vi "Asana_Get.vi"() -> ()   [LabVIEW 2016]
uses:
  <vilib>/httpClient/LabVIEWHTTPClient.lvlib
panel:
  out "Status":string="Idle"
  out "Posting":bool
  out "Body":string="{\"data\":[{\"id\":485255656454849,\"name\":\"Figure out useful API\"},{\"id\":485254540535137,\"name\":\"Figure out useful API\"},{\"id\":483708705076284,\"name\":\"Panther Express Order: CDWG-UPS Battery and Surge protect\"},{\"id\":483695768647078,\"name\":\"Panther Express Order: Grainger - Lascar PS and Scissors\"},{\"id\":483186151754105,\"name\":\"Create a VI that will write a file from a publisher account\"},{\"id\":483194240106048,\"name\":\"Updated CV\"},{\"id\":482695055398718,\"name\":\"Panther Express Order: McMaster - screws, scissors, kapton\"},{\"id\":482610217212443,\"name\":\"Panther Express Order: CDWG-UPS\"},{\"id\":407585611130158,\"name\":\"Damaged items reported in spreadsheet\"},{\"id\":480655848280849,\"name\":\"Panther Express Order: McMaster, Stool for PPMS-DR\"},{\"id\":477959774752493,\"name\":\"Panther Express Order: Grainger stool, etc \"},{\"id\":469638907892082,\"name\":\"QiLi-STO-111-20171024\"},{\"id\":468583209739952,\"name\":\"Panther Express Order: Asylum Research - MFP3D Head Cable\"},{\"id\":466476349857321,\"name\":\"Panther Express Order: Grainger - Roach Kill\"},{\"id\":457225516744036,\"name\":\"Panther Express Order: Grainger - 80/20 Special, Wipers, Tags\"},{\"id\":454524704921360,\"name\":\"Make sure CrystalDiskInfo is running on all of your computers\"},{\"id\":452970255761186,\"name\":\"Panther Express Order: Supra-box, pad, pen, etc\"},{\"id\":450812542170439,\"name\":\"Panther Express Order: B&H, Eneloop 24 batteries \"},{\"id\":446045519104814,\"name\":\"Consider updating your project progress\"},{\"id\":444259581739545,\"name\":\"Panther Express Order: B and H\"},{\"id\":444239318532799,\"name\":\"AsanaBot\"},{\"id\":444214864144911,\"name\":\"Panther Express Order: B and H\"},{\"id\":440454660069823,\"name\":\"Consider updating your project progress\"},{\"id\":439961699416282,\"name\":\"Panther Express Order: Trek Inc \"},{\"id\":439870432141290,\"name\":\"Mapping P/Q as administrator\"},{\"id\":436590367663471,\"name\":\"Read my review of this proposal...\"},{\"id\":437423317842248,\"name\":\"Panther Express Order: CDWG\"},{\"id\":437329183636606,\"name\":\"Panther Express Order: B and H\"},{\"id\":436631000244016,\"name\":\"High-res figures\"},{\"id\":436559576756788,\"name\":\"Review of nature comm paper\"},{\"id\":434949292379141,\"name\":\"Consider updating your project progress\"},{\"id\":431940026570584,\"name\":\"Panther Express Order: Digi-Key\"},{\"id\":431925542819742,\"name\":\"Referee response\"},{\"id\":431034812539576,\"name\":\"Yun-Yi Pai: One-Dimensional Nature of Pairing and Superconductivity at the LaAlO$_3$/SrTiO$_3$ Interface\"},{\"id\":429748551490256,\"name\":\"Panther Express Order: Clark Industry\"},{\"id\":429369274315774,\"name\":\"Consider updating your project progress\"},{\"id\":427825096134432,\"name\":\"Panther Express Order: McMaster\"},{\"id\":427691222436037,\"name\":\"Panther Express Order: Grainger\"},{\"id\":427277290178716,\"name\":\"Panther Express Order: DSS Stockroom\"},{\"id\":426355781160522,\"name\":\"Panther Express Order: McMaster\"},{\"id\":425300320621268,\"name\":\"Panther Express Order: Grainger\"},{\"id\":424594916917454,\"name\":\"Panther Express Order: Grainger\"},{\"id\":423850849835180,\"name\":\"Consider updating your project progress\"},{\"id\":421666010658533,\"name\":\"Panther Express Order: Grainger\"},{\"id\":420450292188130,\"name\":\"Panther Express Order: Count on Tool\"},{\"id\":420274285984926,\"name\":\"Panther Express Order: Supra\"},{\"id\":419973503694738,\"name\":\"A Direct Observation of Room-Temperature Stable Magnetism in LaAlO3/SrTiO3 Heterostructures\"},{\"id\":419007200960117,\"name\":\"Give overview for journal club\"},{\"id\":419211939595159,\"name\":\"Consider updating your project progress\"},{\"id\":418633899494665,\"name\":\"Panther Express Order: Supra\"},{\"id\":418460550035164,\"name\":\"Panther Express Order: Grainger\"},{\"id\":417308065082471,\"name\":\"Pai -- One-Dimensional Nature of Pairing and Superconductivity at the LaAlO$_3$/SrTiO$_3$ Interface\"},{\"id\":417251714966828,\"name\":\"Contact chemarxiv and request removal\"},{\"id\":416724750801660,\"name\":\"Panther Express Order: Digikey\"},{\"id\":416595815316983,\"name\":\"Panther Express Order: CDWG\"},{\"id\":341271010416338,\"name\":\"Leiden CF\"},{\"id\":341271010416342,\"name\":\"PPMS2\"},{\"id\":341271010416340,\"name\":\"MFP3D\"},{\"id\":341701327168967,\"name\":\"Al-SQUID-LAO/STO\"},{\"id\":341701327168968,\"name\":\"1D pairing\"},{\"id\":341271010416334,\"name\":\"Terraces dependence\"},{\"id\":341271010416332,\"name\":\"mK-SPM\"},{\"id\":415394130917359,\"name\":\"Panther Express Order: CDWG\"},{\"id\":415362392608675,\"name\":\"Dying Gallowspole \"},{\"id\":414565496145468,\"name\":\"Panther Express Order: Swagelok\"},{\"id\":414560486678095,\"name\":\"Panther Express Order: PowerTronics\"},{\"id\":414320125293616,\"name\":\"Consider updating your project progress\"},{\"id\":414812763297541,\"name\":\"Backing up Rodia and MFP3D2\"},{\"id\":413707812430964,\"name\":\"Panther Express Order: McMaster\"},{\"id\":412918590813922,\"name\":\"Panther Express Order: Grainger\"},{\"id\":412854250028279,\"name\":\"Panther Express Order: CDWG\"},{\"id\":414812763297546,\"name\":\"Reinstall Rambleon\"},{\"id\":411816952648488,\"name\":\"Panther Express Order: B and H\"},{\"id\":411480040793004,\"name\":\"Panther Express Order: Swagelok\"},{\"id\":411050668817382,\"name\":\"Panther Express Order: Supra\"},{\"id\":410849061822813,\"name\":\"DPC_WATCHDOG_VIOLATION on Windows 10\"},{\"id\":409776701454530,\"name\":\"Panther Express Order: Pfeiffer\"},{\"id\":409725261839576,\"name\":\"Consider updating your project progress\"},{\"id\":408932010835224,\"name\":\"Panther Express Order: Grainger\"},{\"id\":408919683676834,\"name\":\"Panther Express Order: Amazon: Temperhum\"},{\"id\":125608329011186,\"name\":\"order compressed helium\"},{\"id\":407773830393582,\"name\":\"Panther Express Order: LDS Vacuum\"},{\"id\":406802063162283,\"name\":\"UPS Managment and Notification\"},{\"id\":406559591036482,\"name\":\"Panther Express Order: CDWG\"},{\"id\":405460834658478,\"name\":\"Consider updating your project progress\"},{\"id\":404688001223643,\"name\":\"Request for source files: ROPP-100843: \"},{\"id\":403046568483305,\"name\":\"Panther Express Order: B and H\"},{\"id\":240014679645070,\"name\":\"321\"},{\"id\":402248496272499,\"name\":\"From colossal magnetoresistance to solar cells: An overview on 66 years of research into perovskites - Wagner - 2017 - physica status solidi (a) - Wiley Online Library\"},{\"id\":402048376624132,\"name\":\"Panther Express Order: Bluetooth and USB hub\"},{\"id\":402043948639390,\"name\":\"Panther Express Order: Mini-Circuits\"},{\"id\":395892811110536,\"name\":\"Erkut's Visit 2017-08-18\"},{\"id\":400906336596665,\"name\":\"Prospects and Applications Near Ferroelectric Quantum Phase Transitions: A Key Issues Review - IOPscience\"},{\"id\":400863128359472,\"name\":\"Consider updating your project progress\"},{\"id\":400471558989507,\"name\":\"Panther Express Order: Grainger\"},{\"id\":399182657074560,\"name\":\"Post-review modification\"},{\"id\":398583205092188,\"name\":\"Quantized chiral edge conduction on reconfigurable domain walls of a magnetic topological insulator\"},{\"id\":395081310173961,\"name\":\"Panther Express Order: NanoAndMore\"},{\"id\":394425995952756,\"name\":\"Panther Express Order: B and H\"},{\"id\":394147578577517,\"name\":\"Consider updating your project progress\"},{\"id\":393741570332048,\"name\":\"Panther Express Order: Fischer Sci\"},{\"id\":393728961490683,\"name\":\"Panther Express Order: Grainger\"},{\"id\":393425861799391,\"name\":\"Loupe glasses\"},{\"id\":393425861799386,\"name\":\"Humidity Sensor\"},{\"id\":389919070479676,\"name\":\"LED strip\"},{\"id\":392966204577369,\"name\":\"Panther Express Order: Grainger\"},{\"id\":389627825545944,\"name\":\"Consider updating your project progress\"},{\"id\":387484035385757,\"name\":\"Optical routing of TI/STO\"},{\"id\":389052060077622,\"name\":\"[1704.00831] Local optical control of ferromagnetism and chemical potential in a topological insulator\"},{\"id\":387348374446247,\"name\":\"Pai - Present at Group Meeting\"},{\"id\":387264140967807,\"name\":\"Panther Express Order: McMaster\"},{\"id\":385840145696294,\"name\":\"Panther Express Order: McMaster\"},{\"id\":384863397073870,\"name\":\"Consider updating your project progress\"},{\"id\":384334139849136,\"name\":\"Panther Express Order: Hard Drives for Levylab\"},{\"id\":384282457934644,\"name\":\"Panther Express Order: McMaster\"},{\"id\":367057474417733,\"name\":\"New PC (MFP3D)\"},{\"id\":364325321406644,\"name\":\"Document discussing thermal expansion and other issues\"},{\"id\":364325321406641,\"name\":\"Vertical holder for microscope at RT\"},{\"id\":340398386241075,\"name\":\"Isolation Transformer\"},{\"id\":326775992935276,\"name\":\"mK SPM group at ETH\"},{\"id\":321962801394065,\"name\":\"\\\"Matrix box\\\" to filter LEMO signals (black and yellow)\"},{\"id\":378962853779249,\"name\":\"misc\"},{\"id\":344607718799273,\"name\":\"2017-05-17 Skype Meeting\"},{\"id\":248358351003361,\"name\":\"Section 1 - Overview \"},{\"id\":298912981556577,\"name\":\"Nano Letters\"},{\"id\":126345791674174,\"name\":\"Make sure the server is online\"},{\"id\":255953270721811,\"name\":\"Is there a way to configure NaNs get stored as -1?\"},{\"id\":234136524959348,\"name\":\"Gallowspole\"},{\"id\":234136523931720,\"name\":\"PPM2 (Misty)\"},{\"id\":102892368894317,\"name\":\"Coupling to Al SQUIDs (w/ Hatridge)\"},{\"id\":193137962305231,\"name\":\"New PC and PXI\"},{\"id\":174316714177126,\"name\":\"noise in non-contact mode\"},{\"id\":16346183834689,\"name\":\"Videos of how to use MFP3D correctly\"},{\"id\":164934741081297,\"name\":\"Check out and summarize datafinder\"},{\"id\":164713499062215,\"name\":\"Send an Email to Zeldov (this week)\"},{\"id\":5715673502818,\"name\":\"Scanning SET measurements of LAO/STO nanowires w/ Shahal Ilani\"},{\"id\":126345791674164,\"name\":\"Web Services\"},{\"id\":5715673502814,\"name\":\"Nano-SQUID measurements of magnetization and spin currents with Eli Zeldov\"},{\"id\":136636634213865,\"name\":\"Humidity sensing and control outside of the enclosure\"},{\"id\":60311354850707,\"name\":\"SQUID Mask\"},{\"id\":106146774472944,\"name\":\"Writing along and across unit cell steps\"},{\"id\":64122220487809,\"name\":\"Contact Nanomag\"},{\"id\":48971181341219,\"name\":\"Driver for mK AFM\"},{\"id\":15150235906125,\"name\":\"24 to 20 pin adapter\"},{\"id\":49727592364466,\"name\":\"characterize any heating from piezos\"},{\"id\":14977236170882,\"name\":\"Au/LAO/STO Structures\"},{\"id\":383650859418411,\"name\":\"PO:\"},{\"id\":382951012845538,\"name\":\"Panther Express Order: McMaster\"},{\"id\":381019968837796,\"name\":\"Panther Express Order: Digikey\"},{\"id\":379898116941267,\"name\":\"Consider updating your project progress\"},{\"id\":379501609976135,\"name\":\"Panther Express Order: Grainger\"},{\"id\":359337230461679,\"name\":\"Panther Express Order: Grainger Special\"},{\"id\":368042101946896,\"name\":\"Panther Express Order: NanoScience\"},{\"id\":383650859418412,\"name\":\"Review:\"},{\"id\":372506422905539,\"name\":\"PhysRevMaterials.1.011601\"},{\"id\":375791389169587,\"name\":\"Consider updating your project progress\"},{\"id\":373555267523795,\"name\":\"Panther Express Order: Quantum Design\"},{\"id\":372521984820550,\"name\":\"Panther Express Order: Mouser\"},{\"id\":372518137565892,\"name\":\"Panther Express Order: CDWG\"},{\"id\":372517342438507,\"name\":\"Panther Express Order: Grainger\"},{\"id\":372516415483855,\"name\":\"Panther Express Order: Mouser\"},{\"id\":361762437432871,\"name\":\"LSAT\"},{\"id\":371663188737179,\"name\":\"Panther Express Order: McMaster\"},{\"id\":371620557723706,\"name\":\"Cancelled = Panther Express Order: Kurt J. Lesker\"},{\"id\":371224032495043,\"name\":\"Panther Express Order: Mazzella Lifting Technologies\"},{\"id\":370983024120247,\"name\":\"Consider updating your project progress\"},{\"id\":370122582669489,\"name\":\"Panther Express Order: CDWG - Returning\"},{\"id\":370125213842895,\"name\":\"Panther Express Order: CDWG\"},{\"id\":370119572090340,\"name\":\"Panther Express Order: Grainger\"},{\"id\":367760496270952,\"name\":\"Panther Express Order: Grainger\"},{\"id\":367744133364236,\"name\":\"Panther Express Order: DSS Stockroom\"},{\"id\":346485372833056,\"name\":\"Crack in rubber button for putting tip holder\"},{\"id\":365502802890100,\"name\":\"Consider updating your project progress\"},{\"id\":364721085787707,\"name\":\"Panther Express Order: Digikey\"},{\"id\":364658434853254,\"name\":\"Panther Express Order: Mini-Circuits\"},{\"id\":361763253853239,\"name\":\"Chandrasekhar: LSAT/STO (111) MR Hysteresis\"},{\"id\":360092083091940,\"name\":\"Consider updating your project progress\"},{\"id\":359492730923598,\"name\":\"Panther Express Order: International Cryogenics, Inc.\"},{\"id\":359332827077588,\"name\":\"Panther Express Order: Grainger\"},{\"id\":359061921304107,\"name\":\"Panther Express Order: McMaster\"},{\"id\":359056415304435,\"name\":\"Panther Express Order: TREK, INC.\"},{\"id\":358315074302311,\"name\":\"Panther Express Order: Mouser\"},{\"id\":358203951043807,\"name\":\"Panther Express Order: Graingers\"},{\"id\":356484500573696,\"name\":\"Pai - Present at Group Meeting\"},{\"id\":356787632227125,\"name\":\"Panther Express Order: CDW-G\"},{\"id\":356736408768270,\"name\":\"Panther Express Order: Mouser\"},{\"id\":356450795682101,\"name\":\"Pai - Present at Group Meeting\"},{\"id\":355701044972349,\"name\":\"Bigger Local Storage\"},{\"id\":354244206819696,\"name\":\"Consider updating your project progress\"},{\"id\":353860053155370,\"name\":\"Panther Express Order: Grainger\"},{\"id\":352161484261901,\"name\":\"Panther Express Order: McMaster\"},{\"id\":352143249934855,\"name\":\"Panther Express Order: Grainger\"},{\"id\":350033076988687,\"name\":\"Consider updating your project progress\"},{\"id\":344945449319432,\"name\":\"Consider updating your project progress\"},{\"id\":342791884965201,\"name\":\"Beena Kalisky 2017 PRB -2\"},{\"id\":329486926261448,\"name\":\"Beena Kalisky 2017 PRB\"},{\"id\":317228767908080,\"name\":\"https://arxiv.org/pdf/1704.01203.pdf\"},{\"id\":317228767908079,\"name\":\"http://aip.scitation.org/doi/pdf/10.1063/1.4979967\"},{\"id\":341708059341604,\"name\":\"Panther Express Order: Grainger\"},{\"id\":341174718312410,\"name\":\"oxide surfaces\"},{\"id\":340246342866074,\"name\":\"Panther Express Order: CDW-G\"},{\"id\":340174692896356,\"name\":\"Active USB cable\"},{\"id\":337300950631583,\"name\":\"Pai: Intrinsic One-Dimensional Nature of Pairing and Superconductivity at the LaAlO3/SrTiO3 Interface \"},{\"id\":339592127936302,\"name\":\"Consider updating your project progress\"},{\"id\":336723351535456,\"name\":\"Panther Express Order: Grainger\"},{\"id\":334158046623220,\"name\":\"Consider updating your project progress\"},{\"id\":333073854785142,\"name\":\"Panther Express Order: McMaster\"},{\"id\":333047536785694,\"name\":\"Panther Express Order: Fisher Sci.\"},{\"id\":331383475282861,\"name\":\"Pai - Present at Group Meeting\"},{\"id\":330986723902671,\"name\":\"Physics Personality Test\"},{\"id\":329237833123125,\"name\":\"Consider updating your project progress\"},{\"id\":327580444273016,\"name\":\"Panther Express Order: Ideal Vacuum Products\"},{\"id\":326796271040713,\"name\":\"Panther Express Order: Grainger\"},{\"id\":325023011284580,\"name\":\"Panther Express Order: Smartech\"},{\"id\":323356653584989,\"name\":\"Consider updating your project progress\"},{\"id\":322361772416211,\"name\":\"Panther Express Order: Electron Microscopy Sciences\"},{\"id\":318385530450891,\"name\":\"Consider updating your project progress\"},{\"id\":314006257806520,\"name\":\"https://arxiv.org/pdf/1704.00506.pdf\"},{\"id\":314006257806519,\"name\":\"http://aip.scitation.org/doi/full/10.1063/1.4979784\"},{\"id\":314006257806512,\"name\":\"Signatures of unconventional superconductivity in the \\nLaAlO3/SrTiO3 two-dimensional system\"},{\"id\":299178863763963,\"name\":\"LAO/STO(111) SC\"},{\"id\":311980529074688,\"name\":\"Consider updating your project progress\"},{\"id\":310692821032347,\"name\":\"Set up OneDrive desktop sync client on your lab computer\"},{\"id\":309411751793519,\"name\":\"Merge SVN folders?\"},{\"id\":308908236182386,\"name\":\"Drop off Elitebook\"},{\"id\":308582225467303,\"name\":\"Intrinsic One-Dimensional Nature of Pairing and Superconductivity at the LaAlO3/SrTiO3 Interface\"},{\"id\":306812068626788,\"name\":\"Consider updating your project progress\"},{\"id\":305784384153412,\"name\":\"Panther Express Order: LDS Vacuum\"},{\"id\":304104211487255,\"name\":\"Panther Express Order: Edwards Vacuum LLC\"},{\"id\":303070791479196,\"name\":\"A full superconducting dome of strong Ising protection in gated monolayer WS2\"},{\"id\":301428723981105,\"name\":\"Consider updating your project progress\"},{\"id\":300046981186614,\"name\":\"Panther Express Order: Edwards Vacuum LLC\"},{\"id\":299184593375265,\"name\":\"Anisotropic electrical resistance in mesoscopic LaAlO3/SrTiO3 devices with individual domain walls\"},{\"id\":298539775506061,\"name\":\"Panther Express Order: Grainger\"},{\"id\":298481940001964,\"name\":\"Register for PQI2017 poster\"},{\"id\":297595532583898,\"name\":\"First draft of merged document\"},{\"id\":296076631898946,\"name\":\"Consider updating your project progress\"},{\"id\":291976605659177,\"name\":\"Identify five invited speakers\"},{\"id\":290412137790398,\"name\":\"Consider updating your project progress\"},{\"id\":289438637004258,\"name\":\"edge state devices\"},{\"id\":287192304969425,\"name\":\"error\"},{\"id\":284015349878451,\"name\":\"Consider updating your project progress\"},{\"id\":279289670216104,\"name\":\"Consider updating your project progress\"},{\"id\":278428145438049,\"name\":\"Panther Express Order: Newark/element14\"},{\"id\":276973327325408,\"name\":\"Panther Express Order: Thorlabs\"},{\"id\":276592958361938,\"name\":\"paper I mentioned\"},{\"id\":275569092816360,\"name\":\"NSF/NIST interactions - Images\"},{\"id\":274256369094533,\"name\":\"Consider updating your project progress\"},{\"id\":273018357809886,\"name\":\"magnetism in Fe,Sr TiO3\"},{\"id\":273016810148547,\"name\":\"reports on progress of strongly correlated electron systems (to cite)\"},{\"id\":271185183115581,\"name\":\"Panther Express Order: Digi-Key\"},{\"id\":268392008040741,\"name\":\"Consider updating your project progress\"},{\"id\":262737510972781,\"name\":\"Timeline\"},{\"id\":260790785153284,\"name\":\"Consider updating your project progress\"},{\"id\":256547491274555,\"name\":\"Vibration-induced electrical noise in a cryogen-free dilution refrigerator: Characterization, mitigation, and impact on qubit coherence\"},{\"id\":256319557612907,\"name\":\"Radiation pressure excitation of a low temperature atomic force/magnetic force microscope for imaging in 4-300 K temperature range\"},{\"id\":255246756901696,\"name\":\"Consider updating your project progress\"},{\"id\":251781245062089,\"name\":\"add to list of STO-based heterostructures\"},{\"id\":250232403796658,\"name\":\"Consider updating your project progress\"},{\"id\":248358351003360,\"name\":\"Section 6 -Quantum transport in LaAlO3/SrTiO3 nanostructures \"},{\"id\":248358351003359,\"name\":\"Section 5 - Quantum transport in LaAlO3/SrTiO3 heterostructures and microstructures\"},{\"id\":248358351003356,\"name\":\"Section 2 - STO\"},{\"id\":246857701081383,\"name\":\"Panther Express Order: Grainger\"},{\"id\":245350890365818,\"name\":\"Consider updating your project progress\"},{\"id\":244835978480280,\"name\":\"et al. \"},{\"id\":251917656457601,\"name\":\"Pai - Committee Meeting \"},{\"id\":240690315936105,\"name\":\"Purchase Order: Digikey\"},{\"id\":240044916651255,\"name\":\"Verb tense\"},{\"id\":240044916651254,\"name\":\"Topic sentences\"},{\"id\":238607353914986,\"name\":\"Consider updating your project progress\"},{\"id\":238517964498355,\"name\":\"anisotropic magneto-transport of STO\"},{\"id\":238023471615764,\"name\":\"Figure Permission; Caption Formatting\"},{\"id\":205871623279421,\"name\":\"Quantum Transport in LAO/STO nanostructure\"},{\"id\":236625478484745,\"name\":\"Purchase Order: CDW-G\"},{\"id\":236247634432196,\"name\":\"Consider updating your project progress\"},{\"id\":235449330922422,\"name\":\"Pizza 2016-Dec-23\"},{\"id\":234877942816539,\"name\":\"Consider updating your project progress\"},{\"id\":233535709604092,\"name\":\"HousesOfTheHoly\"},{\"id\":234134854974641,\"name\":\"Gallowspole\"},{\"id\":234134854974639,\"name\":\"WindySea\"},{\"id\":233545931129902,\"name\":\"PPM2 (Misty)\"},{\"id\":234134854974637,\"name\":\"Rambleon\"},{\"id\":233535709604088,\"name\":\"HousesOfTheHoly\"},{\"id\":233545934248355,\"name\":\"MFP3D (MFP3D)\"},{\"id\":233533183229280,\"name\":\"citadel-tools\"},{\"id\":233533182880023,\"name\":\"citadel-retro\"},{\"id\":233533182807209,\"name\":\"citadel-lv\"},{\"id\":234134854974633,\"name\":\"Gallowspole\"},{\"id\":234134854974631,\"name\":\"WindySea\"},{\"id\":234136524812777,\"name\":\"WindySea\"},{\"id\":234134854974629,\"name\":\"Rambleon\"},{\"id\":234136524801504,\"name\":\"Rambleon\"},{\"id\":233534097948198,\"name\":\"PPM2 (Misty)\"},{\"id\":233535709604086,\"name\":\"HousesOfTheHoly\"},{\"id\":234136524287242,\"name\":\"HousesOfTheHoly\"},{\"id\":233534100286532,\"name\":\"MFP3D (MFP3D)\"},{\"id\":234136524219653,\"name\":\"MFP3D (MFP3D)\"},{\"id\":234134854974649,\"name\":\"Gallowspole\"},{\"id\":234134854974647,\"name\":\"WindySea\"},{\"id\":234134854974645,\"name\":\"Rambleon\"},{\"id\":234134854974610,\"name\":\"Gallowspole\"},{\"id\":234134854974608,\"name\":\"WindySea\"},{\"id\":234134854974606,\"name\":\"Rambleon\"},{\"id\":232978018888062,\"name\":\"onenote-lv\"},{\"id\":232978018887984,\"name\":\"action-lv\"},{\"id\":233535709604083,\"name\":\"HousesOfTheHoly\"},{\"id\":232978018887979,\"name\":\"MFP3D (MFP3D)\"},{\"id\":232982687193994,\"name\":\"MFP3D (MFP3D)\"},{\"id\":232978018887969,\"name\":\"PPM2 (Misty)\"},{\"id\":232982684401013,\"name\":\"PPM2 (Misty)\"},{\"id\":232521544300963,\"name\":\"ARPES\"},{\"id\":231415486773742,\"name\":\"Consider updating your project progress\"},{\"id\":228562565596800,\"name\":\"Thermodynamic ground states of complex oxide heterointerfaces\"},{\"id\":228562564586949,\"name\":\"Thermodynamic ground states of complex oxide heterointerfaces\"},{\"id\":228388594038088,\"name\":\"Purchase Order: Cryomech\"},{\"id\":227338381758462,\"name\":\"Consider updating your project progress\"},{\"id\":224825092438918,\"name\":\"source drain current inbalance\"},{\"id\":222592455096437,\"name\":\"Consider updating your project progress\"},{\"id\":219282797026522,\"name\":\"paper to cite\"},{\"id\":218797105519435,\"name\":\"Consider updating your project progress\"},{\"id\":214572629093410,\"name\":\"Consider updating your project progress\"},{\"id\":212514588202080,\"name\":\"Create or update research profile for displaywall\"},{\"id\":211609511120715,\"name\":\"Purchase Order: McMaster 1111\"},{\"id\":211606986261980,\"name\":\"Purchase Order: NanoScience\"},{\"id\":211502923267362,\"name\":\"Purchase Order: Grainger\"},{\"id\":210623171573168,\"name\":\"Consider updating your project progress\"},{\"id\":209675948615486,\"name\":\"Create a status update for your project(s)\"},{\"id\":208860928437722,\"name\":\"open browser with ansom.voodoo chrome profile+asana\"},{\"id\":207807821494173,\"name\":\"isotope effect\"},{\"id\":207242673415608,\"name\":\"Time estimate for asana app that lists {project, owner, team, description}?\"},{\"id\":206653597243483,\"name\":\"Consider updating your project progress\"},{\"id\":205871623279426,\"name\":\"3rd meeting\"},{\"id\":205871623279420,\"name\":\"Quantum transport in LAO hetero and microstructure\"},{\"id\":205871623279417,\"name\":\"relevant properties of SrTiO3\"},{\"id\":205329997377261,\"name\":\"set up ansom.voodoo chrome profile for group meeting\"},{\"id\":200724146622861,\"name\":\"Purchase Order: Cryomech\"},{\"id\":198306235896009,\"name\":\"Purchase Order: kensington\"},{\"id\":197716432956347,\"name\":\"Update your user information for new website\"},{\"id\":193769465010869,\"name\":\"Purchase Order: Digikey\"},{\"id\":192498765293369,\"name\":\"Purchase Order: Grainger\"},{\"id\":189507073378549,\"name\":\"Gas Order: PHeN30047 Dry Helium 300 L Grade 4.7\"},{\"id\":189504650003924,\"name\":\"Gas Order: PNiN30040 Dry Nitrogen 300 L Grade 4.0\"},{\"id\":188460139265978,\"name\":\"Issue with references\"},{\"id\":188107077689180,\"name\":\"Pai - Present at Group Meeting\"},{\"id\":186836394912418,\"name\":\"Purchase Order: LDS Vacuum\"},{\"id\":185547258861479,\"name\":\"Purchase Order: Grainger\"},{\"id\":184954848449293,\"name\":\"Check formatting of all references\"},{\"id\":182725168939946,\"name\":\"Another AHE paper\"},{\"id\":180363970686738,\"name\":\"dual gated LAO/STO\"},{\"id\":180199912503203,\"name\":\"Purchase Order: McMaster\"},{\"id\":179675343717938,\"name\":\"Complete information about your PhD committee\"},{\"id\":179602033732027,\"name\":\"oxygen vacancies and magnetism\"},{\"id\":178096297646593,\"name\":\"Register for PQI site\"},{\"id\":174778910265917,\"name\":\"Purchase Order: Cryofab\"},{\"id\":172595123127027,\"name\":\"Permission for figures\"},{\"id\":168638487621070,\"name\":\"Fall availbility for Journal Club/Group Meeting\"},{\"id\":165758900568457,\"name\":\"figure - schematics - (a) ferromagnetism (b) metamagnetism\"},{\"id\":167315771867381,\"name\":\"Purchase Order: Fisher Scientific\"},{\"id\":167312704949565,\"name\":\"Purchase Order: Grainger\"},{\"id\":167302794948722,\"name\":\"Gas Order: PNiN30040 Dry Nitrogen 300 L Grade 4.0\"},{\"id\":165051820720504,\"name\":\"Email to Ariando about hysteresis loops \"},{\"id\":66748281955066,\"name\":\"first draft of manuscript\"},{\"id\":66748281955063,\"name\":\"draft of figures\"},{\"id\":162646311811043,\"name\":\"Review Adv Mat interfacial magnetism manuscript\"},{\"id\":162090010556421,\"name\":\"Identical particle tutorial\"},{\"id\":158715403716316,\"name\":\"Gas Order: PNiN30040 Dry Nitrogen 300 L Grade 4.0\"},{\"id\":158447549681358,\"name\":\"Outline\"},{\"id\":156964267533663,\"name\":\"Restructure the Storyboard Slides\"},{\"id\":156001078337121,\"name\":\"Gas Order: NiLIT240 Liquid Nitrogen 240 L\"},{\"id\":155998596476504,\"name\":\"Gas Order: HeLIT100 Liquid Helium 100 L\"},{\"id\":155998589117385,\"name\":\"Gas Order: HeLIT100 Liquid Helium 100 L\"},{\"id\":155995151009227,\"name\":\"Gas Order: PHeN30047 Dry Helium 300 L Grade 4.7\"},{\"id\":155998056556577,\"name\":\"Gas Order: PNiN30040 Dry Nitrogen 300 L Grade 4.0\"},{\"id\":154818047620897,\"name\":\"2nd Meeting for \\\"Magnetism of Oxide 2DEGs\\\" Review\"},{\"id\":152169474116439,\"name\":\"Gas Order: PNiN30040 Dry Nitrogen 300 L Grade 4.0\"},{\"id\":151532787336380,\"name\":\"fill cold traps\"},{\"id\":150203343351483,\"name\":\"Consider updating your project progress\"},{\"id\":148185352036030,\"name\":\"Purchase Order: McMaster 0624\"},{\"id\":148125603915063,\"name\":\"Purchase Order: CDWG\"},{\"id\":148075035741644,\"name\":\"Gas Order: PNiN30040 Dry Nitrogen 300 L Grade 4.0\"},{\"id\":148075007719819,\"name\":\"Gas Order: PHeN30047 Dry Helium 300 L Grade 4.7\"},{\"id\":147741293752556,\"name\":\"Purchase Order: NanoScience\"},{\"id\":147679797611321,\"name\":\"Purchase Order: Deweyl\"},{\"id\":147539485144755,\"name\":\"Consider updating your project progress\"},{\"id\":146644503148967,\"name\":\"Panther Express Order: digikey\"},{\"id\":145983024360646,\"name\":\"Panther Express Order: CDWG\"},{\"id\":145168997545183,\"name\":\"Leg extender \"},{\"id\":144951255016746,\"name\":\"Consider updating your project progress\"},{\"id\":143654543602587,\"name\":\"Panther Express Order: Grainger\"},{\"id\":142455063150655,\"name\":\"Consider updating your project progress\"},{\"id\":142365294495877,\"name\":\"Cryoclean Mixture\"},{\"id\":140535267769382,\"name\":\"Panther Express Order: CDWG\"},{\"id\":140359819355745,\"name\":\"Panther Express Order: Asylum\"},{\"id\":139697144684082,\"name\":\"Panther Express Order: Thorlabs\"},{\"id\":139625489600022,\"name\":\"Consider updating your project progress\"},{\"id\":139427725339680,\"name\":\"Windows 10 is not compatible with DSC 2013\"},{\"id\":139419703900569,\"name\":\"Panther Express Order: McMaster 0601\"},{\"id\":139321292344178,\"name\":\"6/1/2016 Requestsp\"},{\"id\":137475958858050,\"name\":\"Consider updating your project progress\"},{\"id\":137266598957560,\"name\":\"Panther Express Order: McMaster 0525\"},{\"id\":137234711517004,\"name\":\"New \\\"side\\\" screws for Cantilver holder \"},{\"id\":136656161095434,\"name\":\"fill cold traps\"},{\"id\":135246569001419,\"name\":\"PPMSDR old logfiles to DSC \"},{\"id\":135161713842287,\"name\":\"Consider updating your project progress\"},{\"id\":134230542430553,\"name\":\"Panther Express Order: Fisher Sci.\"},{\"id\":133685066188110,\"name\":\"Panther Express Order: Fisher Sci.\"},{\"id\":133464925727944,\"name\":\"Panther Express Order: Pad2Pad - MFP3D\"},{\"id\":133464903744907,\"name\":\"Panther Express Order: Pad2Pad - Leiden\"},{\"id\":133352726212521,\"name\":\"Gas Order: HeLIT100 Liquid Helium 100 L\"},{\"id\":133352727301064,\"name\":\"Gas Order: HeLIT100 Liquid Helium 100 L\"},{\"id\":133163979281581,\"name\":\"Panther Express Order: McMaster 0513\"},{\"id\":133163336619233,\"name\":\"Panther Express Order: digikey\"},{\"id\":132524671297935,\"name\":\"Consider updating your project progress\"},{\"id\":132289485622195,\"name\":\"Panther Express Order: digikey\"},{\"id\":129697133640053,\"name\":\"Panther Express Order: Grainger\"},{\"id\":129284196867747,\"name\":\"Panther Express Order: McMaster 0506\"},{\"id\":126375051209782,\"name\":\"Create syllabi for your Hardware projects\"},{\"id\":126335696696026,\"name\":\"Identify and update \\\"hardware\\\" projects \"},{\"id\":124643797932692,\"name\":\"Panther Express Order: McMaster 0505\"},{\"id\":124600787822014,\"name\":\"Panther Express Order: Grainger\"},{\"id\":119042115377609,\"name\":\"scanning squid over STO domains\"},{\"id\":118231689016378,\"name\":\"Panther Express Order: LDS Vacuum\"},{\"id\":117776967075898,\"name\":\"Panther Express Order: McMaster 0427\"},{\"id\":116639781688849,\"name\":\"Panther Express Order: digikey\"},{\"id\":116637568666676,\"name\":\"Panther Express Order: LDS Vacuum\"},{\"id\":116062515882754,\"name\":\"Panther Express Order: Kensington \"},{\"id\":113550974735849,\"name\":\"Panther Express Order: digikey\"},{\"id\":113087715702386,\"name\":\"Panther Express Order: McMaster\"},{\"id\":112868661870710,\"name\":\"Panther Express Order: Lesker\"},{\"id\":110615553157182,\"name\":\"Writing test on New Samples processed 20160408\"},{\"id\":110058198031121,\"name\":\"Summary slides and video - Photoconductance and sample batches\"},{\"id\":109789880549867,\"name\":\"Panther Express Order: Grainger\"},{\"id\":108410426618342,\"name\":\"Panther Express Order: McMaster\"},{\"id\":107596056102669,\"name\":\"Gas Order: HeLIT100 Liquid Helium 100 L\"},{\"id\":107405711555654,\"name\":\"Panther Express Order: Lesker\"},{\"id\":106817910671196,\"name\":\"Write report about bad samples from Eom group\"},{\"id\":106015030635433,\"name\":\"Panther Express Order: Mass Vac\"},{\"id\":105760797127891,\"name\":\"Panther Express Order: McMaster\"},{\"id\":105230970347292,\"name\":\"Gas Order: NiLIT240 Liquid Nitrogen 240 L\"},{\"id\":105230957298893,\"name\":\"Gas Order: HeLIT100 Liquid Helium 100 L\"},{\"id\":105230960616871,\"name\":\"Gas Order: HeLIT100 Liquid Helium 100 L\"},{\"id\":103900147761470,\"name\":\"Panther Express Order: International Cryogenics, Inc.\"},{\"id\":103898803921603,\"name\":\"Panther Express Order: McMaster\"},{\"id\":102875955873700,\"name\":\"Gas Order: PHeN30047 Dry Helium 300 L Grade 4.7\"},{\"id\":102875954228671,\"name\":\"Panther Express Order: Grainger\"},{\"id\":99793396757939,\"name\":\"Write 5 questions you think someone might ask about your talk\"},{\"id\":97940291550907,\"name\":\"Panther Express Order: Grainger\"},{\"id\":97644768510106,\"name\":\"Identify five invited speakers\"},{\"id\":97637468148862,\"name\":\"Make cover slide uniform\"},{\"id\":97637139955722,\"name\":\"Make cover slide uniform\"},{\"id\":97139690926207,\"name\":\"Panther Express Order: digikey\"},{\"id\":97100330896667,\"name\":\"Panther Express Order: Replacement computer for Levylab's OCEAN\"},{\"id\":97007676080216,\"name\":\"Panther Express Order: Grainger\"},{\"id\":96477683751693,\"name\":\"Gas Order: NiLIT240 Liquid Nitrogen 240 L\"},{\"id\":96475095186333,\"name\":\"Gas Order: HeLIT100 Liquid Helium 100 L\"},{\"id\":96010421506370,\"name\":\"Panther Express Order: LDS Vacuum\"},{\"id\":95771399392397,\"name\":\"Make sure that Munir insured our Leiden Insert\"},{\"id\":94279700915749,\"name\":\"Panther Express Order: Swagelok\"},{\"id\":93508225747564,\"name\":\"Purchase Order: McMaster II\"},{\"id\":93888861428105,\"name\":\"Initial conductance check\"},{\"id\":93298331967261,\"name\":\"Purchase Order: McMaster\"},{\"id\":92517652641644,\"name\":\"Gas Order: NiLIT240 Liquid Nitrogen 240 L\"},{\"id\":92517646979979,\"name\":\"Gas Order: HeLIT100 Liquid Helium 100 L\"},{\"id\":92517641415715,\"name\":\"Gas Order: HeLIT100 Liquid Helium 100 L\"},{\"id\":92514749657013,\"name\":\"Gas Order: HeLIT100 Liquid Helium 100 L\"},{\"id\":92514746540326,\"name\":\"Gas Order: HeLIT100 Liquid Helium 100 L\"},{\"id\":92511765586960,\"name\":\"Gas Order: PHeN30047 Dry Helium 300 L Grade 4.7\"},{\"id\":91035101636666,\"name\":\"Dengyu Yang\"},{\"id\":89996309650619,\"name\":\"Gas Order: HeLIT100 Liquid Helium 100 L\"},{\"id\":89996264569424,\"name\":\"Gas Order: HeLIT100 Liquid Helium 100 L\"},{\"id\":89444296728938,\"name\":\"Panther Express Order: Graingers\"},{\"id\":89140667028878,\"name\":\"Gas Order: NiLIT240 Liquid Nitrogen 240 L\"},{\"id\":87072441086417,\"name\":\"Unlabeled Gas Tanks\"},{\"id\":87072441086407,\"name\":\"Secure Gas Tanks\"},{\"id\":85849392920710,\"name\":\"Gas Order: NiLIT240 Liquid Nitrogen 240 L\"},{\"id\":85439088878414,\"name\":\"Gas Order: HeLIT100 Liquid Helium 100 L\"},{\"id\":85439071294142,\"name\":\"Gas Order: HeLIT100 Liquid Helium 100 L\"},{\"id\":85439074512744,\"name\":\"Gas Order: HeLIT100 Liquid Helium 100 L\"},{\"id\":85438425249668,\"name\":\"Gas Order: HeLIT100 Liquid Helium 100 L\"},{\"id\":82832751834024,\"name\":\"Pai - Record offline presentations\"},{\"id\":79517035865800,\"name\":\"Availability for undergrad group meeting\"},{\"id\":79183424564909,\"name\":\"Panther Express Order: DSS Stockroom\"},{\"id\":79035356733892,\"name\":\"DSC Tutorial for First Experience Undergrads\"},{\"id\":78914474708486,\"name\":\"Gas Order: PHeN30047 Dry Helium 300 L Grade 4.7\"},{\"id\":78914468031217,\"name\":\"Gas Order: PHeN30047 Dry Helium 300 L Grade 4.7\"},{\"id\":78878779991836,\"name\":\"Gas Order: HeLIT100 Liquid Helium 100 L\"},{\"id\":78878776698753,\"name\":\"Gas Order: HeLIT100 Liquid Helium 100 L\"},{\"id\":67901183843210,\"name\":\"Template 2016\"},{\"id\":76984015749210,\"name\":\"Gas Order: HeLIT100 Liquid Helium 100 L\"},{\"id\":76984015562239,\"name\":\"Gas Order: HeLIT100 Liquid Helium 100 L\"},{\"id\":75270418081803,\"name\":\"Gas Order: HeLIT100 Liquid Helium 100 L\"},{\"id\":75270536372552,\"name\":\"Gas Order: HeLIT100 Liquid Helium 100 L\"},{\"id\":75269737496800,\"name\":\"Gas Order: NiLIT240 Liquid Nitrogen 240 L\"},{\"id\":75269733577111,\"name\":\"Gas Order: PHeN30047 Dry Helium 300 L Grade 4.7\"},{\"id\":75269732850731,\"name\":\"Gas Order: PHeN30047 Dry Helium 300 L Grade 4.7\"},{\"id\":71558202092309,\"name\":\"Gas Order: HeLIT100 Liquid Helium 100 L\"},{\"id\":71556340730120,\"name\":\"Gas Order: HeLIT100 Liquid Helium 100 L\"},{\"id\":71546087940685,\"name\":\"Gas Order: HeLIT100 Liquid Helium 100 L\"},{\"id\":71342381458839,\"name\":\"Gas Order: HeLIT100 Liquid Helium 100 L\"},{\"id\":70505084073015,\"name\":\"Artificial Atoms Based on Correlated Materials\"},{\"id\":70594034101133,\"name\":\"IVC - Still Leak\"},{\"id\":70360131285912,\"name\":\"Gas Order: HeLIT100 Liquid Helium 100 L\"},{\"id\":69517290878209,\"name\":\"Gas Order: HeLIT100 Liquid Helium 100 L\"},{\"id\":69517279337066,\"name\":\"Gas Order: NiLIT240 Liquid Nitrogen 240 L\"},{\"id\":69380475681032,\"name\":\"Noise 2015-11-28\"},{\"id\":69353153527219,\"name\":\"Panther Express Order: DSS Stockroom\"},{\"id\":68692401733271,\"name\":\"Gas Order: NiLIT240 Liquid Nitrogen 240 L\"},{\"id\":68477888191438,\"name\":\"Gas Order: HeLIT100 Liquid Helium 100 L\"},{\"id\":68477883175783,\"name\":\"Gas Order: HeLIT100 Liquid Helium 100 L\"},{\"id\":67415569223954,\"name\":\"Gas Order: NiLIT240 Liquid Nitrogen 240 L\"},{\"id\":67415531566908,\"name\":\"Gas Order: PHeN30047 Dry Helium 300 L Grade 4.7\"},{\"id\":67415524795761,\"name\":\"Gas Order: PNiN30040 Dry Nitrogen 300 L Grade 4.0\"},{\"id\":66572876306298,\"name\":\"Gas Order: HeLIT100 Liquid Helium 100 L\"},{\"id\":66564591185969,\"name\":\"IVC Pressure Anomaly \"},{\"id\":65922131372281,\"name\":\"Active Group Calendar (Calendar ID: ansom.voodoo@levylab.org)?\"},{\"id\":64759885620033,\"name\":\"What is current status of PPMS2?\"},{\"id\":64365385628585,\"name\":\"Gas Order: HeLIT100 Liquid Helium 100 L\"},{\"id\":62813684944748,\"name\":\"Gas Order: HeLIT100 Liquid Helium 100 L\"},{\"id\":60347878452011,\"name\":\"Identify \\\"Critical\\\" machines\"},{\"id\":60693774267114,\"name\":\"Gas Order: HeLIT100 Liquid Helium 100 L\"},{\"id\":60693447855440,\"name\":\"Panther Express Order: ANOTOP Syringe Filters by Whatman 10/0.02 S 50/PK\"},{\"id\":60623045798315,\"name\":\"Gas Order: NiLIT240 Liquid Nitrogen 240 L\"},{\"id\":59092063781082,\"name\":\"Gas Order: PHeN30047 Dry Helium 300 L Grade 4.7\"},{\"id\":58922703953013,\"name\":\"LaAlO3/SrTiO3 FIELD EFFECT NANODEVICES USING IN-SITU GROWN AU TOP GATES\"},{\"id\":58020547330539,\"name\":\"Gas Order: HeLIT100 Liquid Helium 100 L\"},{\"id\":55741637918671,\"name\":\"Gas Order: HeLIT100 Liquid Helium 100 L\"},{\"id\":54965008246752,\"name\":\"Virus concern for PPMS2 PC\"},{\"id\":49772222616415,\"name\":\"research low temperature fiber-fiber connection\"},{\"id\":53179741069779,\"name\":\"fiber splicer\"},{\"id\":52981132388882,\"name\":\"Gas Order: NiLIT240 Liquid Nitrogen 240 L\"},{\"id\":52981130972308,\"name\":\"Gas Order: ordered 2\"},{\"id\":52960073478945,\"name\":\"Video Colleciton\"},{\"id\":52912076187742,\"name\":\"Get Profile Picture Retaken\"},{\"id\":51337574061117,\"name\":\"Gas Order: HeLIT100 Liquid Helium 100 L\"},{\"id\":51337572535519,\"name\":\"Gas Order: HeLIT60 Liquid Helium 60 L\"},{\"id\":49985126663583,\"name\":\"fusion splicer\"},{\"id\":47475245341229,\"name\":\"PPMS1 Video Collection\"},{\"id\":47228951878840,\"name\":\"Gas Order: NiLIT240 Liquid Nitrogen 240 L\"},{\"id\":47228948073557,\"name\":\"Gas Order: HeLIT60 Liquid Helium 60 L\"},{\"id\":46813161714986,\"name\":\"Recording 2015-08-25\"},{\"id\":46665024978875,\"name\":\"Pai\"},{\"id\":46451237981190,\"name\":\"Lacie Drive\"},{\"id\":46481165940621,\"name\":\"Gas Order: HeLIT60 Liquid Helium 60 L\"},{\"id\":46324425788083,\"name\":\"Select a location\"},{\"id\":45894530053709,\"name\":\"Usage Report\"},{\"id\":45772632052935,\"name\":\"Gas Order: NiLIT240 Liquid Nitrogen 240 L\"},{\"id\":45772484755111,\"name\":\"Gas Order: HeLIT60 Liquid Helium 60 L\"},{\"id\":45772425656128,\"name\":\"Gas Order: PHeN30047 Dry Helium 300 L Grade 4.7\"},{\"id\":44950377136983,\"name\":\"Email Malwarebytes License Key (PPMS2)\"},{\"id\":44909478056165,\"name\":\"WEB SERVICES\"},{\"id\":44672135481298,\"name\":\"Advanced Plotting Toolkit of LabVIEW?\"},{\"id\":44459146917824,\"name\":\"How to handle string-based variables?\"},{\"id\":44383550932019,\"name\":\"Add button to make y scales the same\"},{\"id\":44390960900210,\"name\":\"Gas Order: NiLIT240 Liquid Nitrogen 240 L\"},{\"id\":42039043355296,\"name\":\"MFP3D SOCKET CONNECTION\"},{\"id\":44190505500126,\"name\":\"database.vi export data\"},{\"id\":43568314688959,\"name\":\"Gas Order: HeLIT60 Liquid Helium 60 L\"},{\"id\":43568318523305,\"name\":\"Gas Order: HeLIT60 Liquid Helium 60 L\"},{\"id\":43498782106627,\"name\":\"Gas Order: NiLIT240 Liquid Nitrogen 240 L\"},{\"id\":43133366524529,\"name\":\"Panther Express Order: Door latch for MFP3D\"},{\"id\":43017916888398,\"name\":\"Door Draw Latch\"},{\"id\":42802469755967,\"name\":\"Gas Order: HeLIT100 Liquid Helium 100 L\"},{\"id\":42802481493325,\"name\":\"Gas Order: HeLIT60 Liquid Helium 60 L\"},{\"id\":42607888722506,\"name\":\"Gas Order: PHeN30047 Dry Helium 300 L Grade 4.7\"},{\"id\":42361914774494,\"name\":\"PPMS2 Pai\"},{\"id\":41868342016935,\"name\":\"housesoftheholy \\\"crash\\\"\"},{\"id\":41857149230531,\"name\":\"Buy new hose for LN2 \"},{\"id\":40666117647959,\"name\":\"Summary slides for VESFET project\"},{\"id\":40547911808045,\"name\":\"Nitrogen Fill\"},{\"id\":40547911808043,\"name\":\"Helium Fill\"},{\"id\":40466768196523,\"name\":\"Return Krohn-Hite amplifier\"},{\"id\":40122617706426,\"name\":\"Possible Impedance Line Blockage\"},{\"id\":40086998767434,\"name\":\"PPMS2 Reservation System now online\"},{\"id\":39917242962802,\"name\":\"Wire Bonder Experience\"},{\"id\":39819206178756,\"name\":\"Training Syllabus\"},{\"id\":39774654317576,\"name\":\"Register as a Panther Express Shopper\"},{\"id\":39655102938145,\"name\":\"PPMS2 + PPMS1 Helium Recovery Log\"},{\"id\":39442085421999,\"name\":\"Purchase Order: Tweezers for MFP-3D\"},{\"id\":39442158435246,\"name\":\"Purchase Order: Scribers for MFP3D and Cypher\"},{\"id\":39572885646013,\"name\":\"PPMS2 User Log\"},{\"id\":33342763564118,\"name\":\"Purchase Order: Dewyle\"},{\"id\":38138004176756,\"name\":\"add 2nd connection for dewar boiloff 2nd floor\"},{\"id\":35017879873994,\"name\":\"Magneto-transport study of top- and back-gated LaAlO3/SrTiO3 heterostructures\"},{\"id\":34623701744210,\"name\":\"Bad Points\"},{\"id\":34524190195189,\"name\":\"Quotes and PO\"},{\"id\":32469359569159,\"name\":\"PPMS1\"},{\"id\":32469359569163,\"name\":\"THz\"},{\"id\":33880566013029,\"name\":\"Tracking no. 773614658330\"},{\"id\":33880566013023,\"name\":\"Packaging \"},{\"id\":33694543212846,\"name\":\"RMA\"},{\"id\":32583443727807,\"name\":\"Cypher Problems? \"},{\"id\":32531733315515,\"name\":\"Kerr Experiment - Laser \"},{\"id\":32391720514289,\"name\":\"PPMS2\"},{\"id\":32144025616482,\"name\":\"arxiv.org/pdf/1504.04226.pdf\"},{\"id\":31535553536336,\"name\":\"Report: \"},{\"id\":23720573266139,\"name\":\"Highest Priority:\"},{\"id\":15341145574862,\"name\":\"Candidacy Requirements \"},{\"id\":31535553536327,\"name\":\"Laser Diode\"},{\"id\":31535553536325,\"name\":\"Streaks, noises in scans\"},{\"id\":31530102907533,\"name\":\"Identify systems\"},{\"id\":25765815716380,\"name\":\"Create new ppt template\"},{\"id\":25049451790340,\"name\":\"error in 'write_18T_Data_to_DSC.vi'\"},{\"id\":25062154349101,\"name\":\"Flagged Inbox messages\"},{\"id\":23720573266138,\"name\":\"TEST\"},{\"id\":23444437164615,\"name\":\"FP logfiles to DSC\"},{\"id\":23444437164608,\"name\":\"FP logfiles\"},{\"id\":23208496995936,\"name\":\"X-Ray Diffraction\"},{\"id\":23171626185571,\"name\":\"Yun-Yi Pai\"},{\"id\":22958487398402,\"name\":\"Problem reading variable\"},{\"id\":21282009632622,\"name\":\"VI that comments on Asana\"},{\"id\":20932767600014,\"name\":\"Database.vi\"},{\"id\":14434592387491,\"name\":\"Temperhum SCADA-enabled project\"},{\"id\":20121100611243,\"name\":\"Join APS\"},{\"id\":16050071994557,\"name\":\"\"},{\"id\":15694070462367,\"name\":\"Yun-Yi Pai\"},{\"id\":16031545542630,\"name\":\"Figure out useful API\"},{\"id\":15587748171046,\"name\":\"Let me know your requirements for file uploads\"},{\"id\":15281311128973,\"name\":\"PXI chassis/controller/4461 card\"},{\"id\":15490566998827,\"name\":\"Friday Aug 22 8:30-4:30 JW Connolly ballroom in Alumni Hall.\"},{\"id\":15490267999932,\"name\":\"Wednesday Aug 20 12PM-3PM Orientation, 9 floor, LRDC\\n\"},{\"id\":15490267999926,\"name\":\"Wednesday Aug 20 9AM Departmental Pretest 300 OEH \\n\"},{\"id\":15490267999928,\"name\":\"Friday Aug 15 1PM Car maintenance\"},{\"id\":15345453519541,\"name\":\"Evaluate LabVIEW 2014 and DSC 2014\"},{\"id\":15281311128985,\"name\":\"Connect electric cables GHS to Fridge\"},{\"id\":15490267999922,\"name\":\"Friday Aug 15 10AM  TA English screening\"},{\"id\":15281311128963,\"name\":\"MNK Electronics\"},{\"id\":12922787870856,\"name\":\"Track the form from OIS to Cornell\"},{\"id\":13226816508508,\"name\":\"LabView for Oxford Power Supply IPS (Pai)\"},{\"id\":12619497892724,\"name\":\"Get clean shoes\"},{\"id\":12619497892725,\"name\":\"Join Asana groups (coffee, instruments, etc)\"},{\"id\":12619497892726,\"name\":\"Computer 101 (e.g., voodoo, passwords, )\"},{\"id\":12619497892730,\"name\":\"Set up onedrive account\"},{\"id\":12619497892731,\"name\":\"Create onenote notebook on voodoo\"},{\"id\":12619497892748,\"name\":\"Overview/assignment of research projects\"},{\"id\":13399982349813,\"name\":\"Pai\"},{\"id\":14403537138063,\"name\":\"Pai\"},{\"id\":14828153676801,\"name\":\"Pai\"},{\"id\":15206586326300,\"name\":\"Pai\"},{\"id\":15745773221705,\"name\":\"Pai\"},{\"id\":16054912372636,\"name\":\"Pai\"},{\"id\":16393856754839,\"name\":\"Pai\"},{\"id\":17267863198360,\"name\":\"Pai\"},{\"id\":18284802066418,\"name\":\"Pai\"},{\"id\":19639779663679,\"name\":\"Pai\"},{\"id\":20403526778521,\"name\":\"Pai\"},{\"id\":22451973230355,\"name\":\"Pai\"},{\"id\":24626000123341,\"name\":\"Pai\"},{\"id\":13444665969774,\"name\":\"Make calibration files for magnet sensors\"},{\"id\":25036467465063,\"name\":\"Au/LAO/STO\"},{\"id\":14519968107958,\"name\":\"VI that Sends Email (Pai)\"},{\"id\":12922787870858,\"name\":\"Handling Error of VRM (Pai)\"},{\"id\":14519968107971,\"name\":\"VI that Tweets (Pai)\"},{\"id\":14519968107967,\"name\":\"Triangle Wave in the VI (Pai)\"},{\"id\":14705126625676,\"name\":\"Setting up Oral Comprehensive Exam (Pai)\"},{\"id\":14705562644141,\"name\":\"LabVIEW: temperature log reader (originally network-shared variable)  (Pai)\"},{\"id\":14799656824416,\"name\":\"LabVIEW: Network Published Variable (Pai)\"},{\"id\":24233115328645,\"name\":\"Measurements\"},{\"id\":24233115328641,\"name\":\"Writing Practice\"},{\"id\":31535553536341,\"name\":\"Not-so-active:\"},{\"id\":20121100611235,\"name\":\"LaAlO$_3$/SrTiO$_3$ fieldH-effect nanodevices using in-situ-grown Au top gates\"},{\"id\":31243749100437,\"name\":\"LaAlO$_3$/SrTiO$_3$ fieldH-effect nanodevices using in-situ-grown Au top gates\"},{\"id\":12619497892747,\"name\":\"labview tutorials\"},{\"id\":14519968107953,\"name\":\"Mains Noise in the Lock-In (Pai)\"},{\"id\":15184861713797,\"name\":\"LabVIEW-OneNote Integration \"},{\"id\":15227068197779,\"name\":\"Integrate Lithography with DSC\"},{\"id\":12619497892733,\"name\":\"Instrument Training\"},{\"id\":13401135687112,\"name\":\"SCADA Architecture\"},{\"id\":15318023363845,\"name\":\"Add sound insulation to Pulse Tube and Hoses\"},{\"id\":31535553536340,\"name\":\"Group Meeting:\"},{\"id\":23363566637297,\"name\":\"Pai\"},{\"id\":26039795368668,\"name\":\"Pai\"},{\"id\":30933479854041,\"name\":\"Pai\"},{\"id\":32126911094335,\"name\":\"Pai\"},{\"id\":33123639996005,\"name\":\"Pai\"},{\"id\":34780416364185,\"name\":\"Pai\"},{\"id\":38079461639187,\"name\":\"Pai\"},{\"id\":54496335572974,\"name\":\"Pai\"},{\"id\":55465016700407,\"name\":\"Pai\"},{\"id\":57166418391441,\"name\":\"Pai\"},{\"id\":69703354972979,\"name\":\"Pai\"},{\"id\":75191679779490,\"name\":\"Pai\"},{\"id\":82791323231698,\"name\":\"Pai - Present at Group Meeting\"},{\"id\":60716308241475,\"name\":\"Reformat slides for NRI talk\"},{\"id\":55028657177022,\"name\":\"Pai: Vertical gating of sketched nanodevices\"},{\"id\":79053344506023,\"name\":\"Research overview video\"},{\"id\":85098350325171,\"name\":\"Pai - Record offline presentations\"},{\"id\":87672317326778,\"name\":\"Pai - Present at Group Meeting\"},{\"id\":91803731546959,\"name\":\"Pai - Present at Group Meeting\"},{\"id\":94675143972847,\"name\":\"Pai - Present at Group Meeting\"},{\"id\":104733336856616,\"name\":\"Pai - Present at Group Meeting\"},{\"id\":104738335766106,\"name\":\"Pai - Present at Group Meeting\"},{\"id\":104741122743423,\"name\":\"Pai - Present at Group Meeting\"},{\"id\":104749904874761,\"name\":\"Pai - Present at Group Meeting\"},{\"id\":106987042992057,\"name\":\"Pai - Present at Group Meeting\"},{\"id\":111610280176560,\"name\":\"Email video to Wisconsin\"},{\"id\":110084654556083,\"name\":\"Pai - Present at Group Meeting\"},{\"id\":112969362201807,\"name\":\"Pai - Present at Group Meeting\"},{\"id\":118377479879577,\"name\":\"Pai - Present at Group Meeting\"},{\"id\":119753237007555,\"name\":\"Pai - Present at Group Meeting\"},{\"id\":132422692346271,\"name\":\"Pai - Present at Group Meeting\"},{\"id\":134318049980734,\"name\":\"Pai - Present at Group Meeting\"},{\"id\":138816041439245,\"name\":\"Pai - Present at Group Meeting\"},{\"id\":138822922653099,\"name\":\"Pai - Present at Group Meeting\"},{\"id\":144235850055093,\"name\":\"Pai - Present at Group Meeting\"},{\"id\":142364919502684,\"name\":\"fill cold traps\"},{\"id\":144237743380951,\"name\":\"Pai - Present at Group Meeting\"},{\"id\":145848250620244,\"name\":\"fill cold traps\"},{\"id\":149337353454267,\"name\":\"Pai - Present at Group Meeting\"},{\"id\":148966498582465,\"name\":\"fill cold traps\"},{\"id\":149344610922992,\"name\":\"Pai - Present at Group Meeting\"},{\"id\":154419569455436,\"name\":\"Pai - Present at Group Meeting\"},{\"id\":153774104497474,\"name\":\"fill cold traps\"},{\"id\":154435052614206,\"name\":\"Pai - Present at Group Meeting\"},{\"id\":157193941228717,\"name\":\"Pai - Present at Group Meeting\"},{\"id\":158874735863023,\"name\":\"fill cold traps\"},{\"id\":162773842739830,\"name\":\"Pai - Present at Group Meeting\"},{\"id\":161819711491200,\"name\":\"fill cold traps\"},{\"id\":164494864499975,\"name\":\"Pai - Present at Group Meeting\"},{\"id\":165695525848377,\"name\":\"Pai - Present at Group Meeting\"},{\"id\":168595517948863,\"name\":\"Pai - Present at Group Meeting\"},{\"id\":171809862588006,\"name\":\"Pai - Present at Group Meeting\"},{\"id\":177049197108474,\"name\":\"Pai - Present at Group Meeting\"},{\"id\":177079031119398,\"name\":\"Pai - Present at Group Meeting\"},{\"id\":181040801835513,\"name\":\"Pai - Present at Group Meeting\"},{\"id\":184070060075469,\"name\":\"Pai - Present at Group Meeting\"},{\"id\":191580029391855,\"name\":\"Pai - Present at Group Meeting\"},{\"id\":194771548805693,\"name\":\"Pai - Present at Group Meeting\"},{\"id\":198392446277516,\"name\":\"Pai - Present at Group Meeting\"},{\"id\":205560566546403,\"name\":\"Pai - Present at Group Meeting\"},{\"id\":196925435070120,\"name\":\"Pai - $LaAlO_3/SrTiO_3$--A Tale of Two Magnetisms\"},{\"id\":205575904654313,\"name\":\"Pai - Present at Group Meeting\"},{\"id\":209247659427764,\"name\":\"Pai - Present at Group Meeting\"},{\"id\":213128986302479,\"name\":\"Pai - Present at Group Meeting\"},{\"id\":217625595212760,\"name\":\"Pai - Present at Group Meeting\"},{\"id\":230039719086632,\"name\":\"Pai - Present at Group Meeting\"},{\"id\":230039750281876,\"name\":\"Pai - Present at Group Meeting\"},{\"id\":230055619450346,\"name\":\"Pai - Present at Group Meeting\"},{\"id\":237102956730719,\"name\":\"Pai - Present at Group Meeting\"},{\"id\":237104530895739,\"name\":\"Pai - Present at Group Meeting\"},{\"id\":237104520835462,\"name\":\"Pai - Present at Group Meeting\"},{\"id\":242979742068291,\"name\":\"Pai - Present at Group Meeting\"},{\"id\":253411870083341,\"name\":\"Pai - Present at Group Meeting\"},{\"id\":253413104460047,\"name\":\"Pai - Present at Group Meeting\"},{\"id\":258717138345560,\"name\":\"Pai - Present at Group Meeting\"},{\"id\":272650480868050,\"name\":\"Pai - Present at Group Meeting\"},{\"id\":272685390854937,\"name\":\"Pai - Present at Group Meeting\"},{\"id\":277151459045772,\"name\":\"Pai - Present at Group Meeting\"},{\"id\":282337242534980,\"name\":\"Pai - Present at Group Meeting\"},{\"id\":304791318702765,\"name\":\"Pai - Present at Group Meeting\"},{\"id\":304802683792269,\"name\":\"Pai - Present at Group Meeting\"},{\"id\":304806896322522,\"name\":\"Pai - Present at Group Meeting\"},{\"id\":304834760103838,\"name\":\"Pai - Present at Group Meeting\"},{\"id\":310506698372899,\"name\":\"Pai - Present at Group Meeting\"},{\"id\":316802126797194,\"name\":\"Pai - Present at Group Meeting\"},{\"id\":320667637363535,\"name\":\"Pai - Present at Group Meeting\"},{\"id\":331412844306639,\"name\":\"Pai - Present at Group Meeting\"},{\"id\":338715892444338,\"name\":\"Pai - Present at Group Meeting\"},{\"id\":342941227852313,\"name\":\"Pai - Present at Group Meeting\"},{\"id\":349715879531905,\"name\":\"Pai - Present at Group Meeting\"},{\"id\":367587459629721,\"name\":\"Pai - Present at Group Meeting\"},{\"id\":367654486705575,\"name\":\"Pai - Present at Group Meeting\"},{\"id\":377766792027523,\"name\":\"Pai - Present at Group Meeting\"},{\"id\":36028106051324,\"name\":\"One-Dimensional Nature of Pairing and Superconductivity at the LaAlO3/SrTiO3 Interface\"},{\"id\":377841647017700,\"name\":\"Pai - Present at Group Meeting\"},{\"id\":381874355549157,\"name\":\"Pai - Present at Group Meeting\"},{\"id\":387348407046378,\"name\":\"Pai - Present at Group Meeting\"},{\"id\":391617386026136,\"name\":\"Pai - Present at Group Meeting\"},{\"id\":397242153900879,\"name\":\"Pai - Present at Group Meeting\"},{\"id\":403758478732996,\"name\":\"Pai - Present at Group Meeting\"},{\"id\":407264827347577,\"name\":\"Pai - Present at Group Meeting\"},{\"id\":411597923197262,\"name\":\"Pai - Present at Group Meeting\"},{\"id\":416303545845913,\"name\":\"Pai - Present at Group Meeting\"},{\"id\":428875800618091,\"name\":\"Pai - Present at Group Meeting\"},{\"id\":428876791415287,\"name\":\"Pai - Present at Group Meeting\"},{\"id\":436546621361853,\"name\":\"Pai - Present at Group Meeting\"},{\"id\":440011240699734,\"name\":\"Pai - Present at Group Meeting\"},{\"id\":451135334407500,\"name\":\"Pai - Present at Group Meeting\"},{\"id\":451135334407510,\"name\":\"Pai - Present at Group Meeting\"},{\"id\":451177454750752,\"name\":\"Pai - Present at Group Meeting\"},{\"id\":457132355283245,\"name\":\"Pai - Present at Group Meeting\"},{\"id\":468525661428301,\"name\":\"Pai - Present at Group Meeting\"},{\"id\":468653439236876,\"name\":\"Pai - Present at Group Meeting\"},{\"id\":480637847303207,\"name\":\"Pai - Present at Group Meeting\"},{\"id\":480715171118440,\"name\":\"Pai - Present at Group Meeting\"}]}"
  out "Headers":string="HTTP/1.1 200 OK\r\nServer: nginx\r\nDate: Tue, 21 Nov 2017 16:40:08 GMT\r\nContent-Type: application/json; charset=UTF-8\r\nTransfer-Encoding: chunked\r\nConnection: keep-alive\r\nX-Asana-Api-Version: 1.1\r\nX-Asana-Preferred-Release-Revision: 20171120_221241_867ba3e15db2221bfc1a505ff00d5822edf28beb\r\nX-Robots-Tag: none\r\nStrict-Transport-Security: max-age=31536000; includeSubDomains\r\nDatacenter-Time-End: 1511282408.495\r\nX-LoadBalancer: prod-lb000.ec2\r\n\r\n"
  # "Direction:\nType in the partial name of the section \nto search, run the VI, and the Section ID\nwill be returned after the HTTP request\nis completed. This could take 3 - 30 sec."
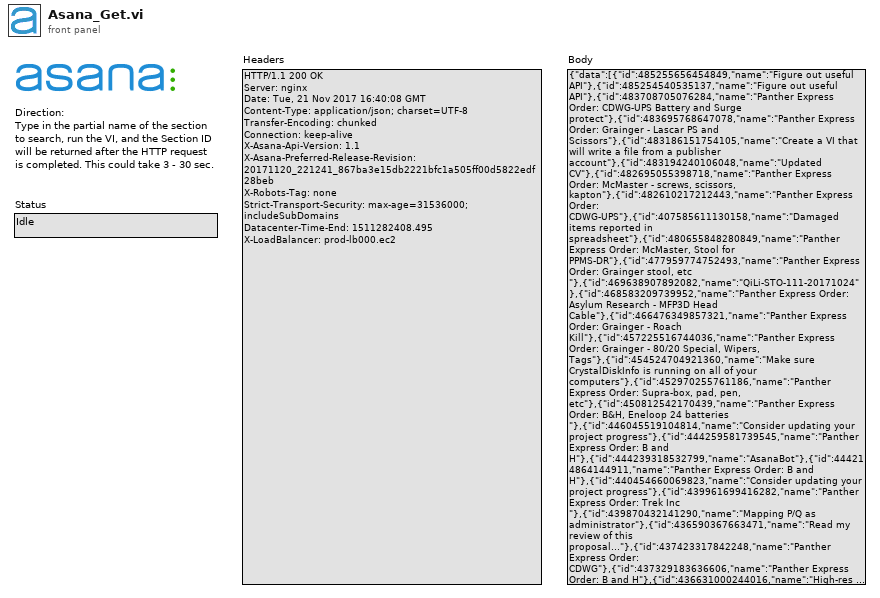
[diagram p1: front panel]
types:
  T1 = typedef "LabVIEWHTTPClient.lvlib/ClientHandle.ctl" = refnum<k1>
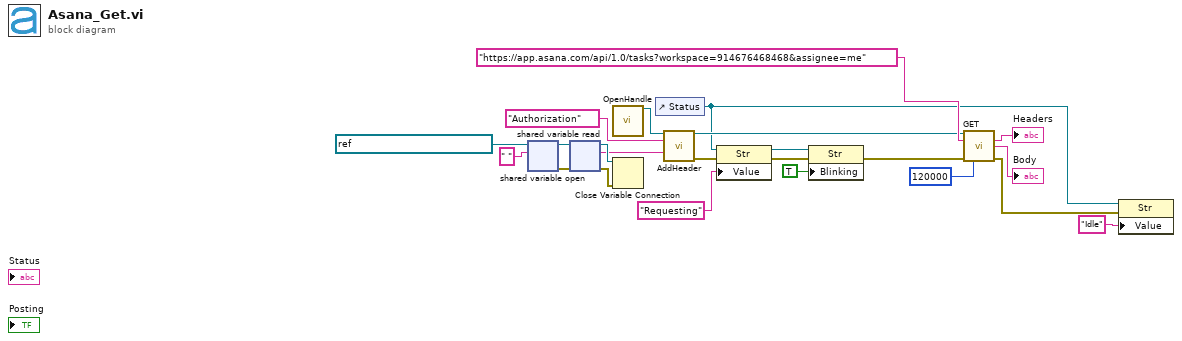
[diagram p0: block diagram]
diagram:
  n1 = shared-variable-open(refnum<k21> "ni.var.psp://housesoftheholy/OneNote API HTTP/Asana Access Token 15669051163913" ("shared variable refnum in"), " " ("string")) -> (w16:refnum<k21>, w15:errorcluster)  [unwired: 2 in]
  n2 = shared-variable-read(w16, w15) -> (w14:refnum<k21>, w13:errorcluster, w12:string)  [unwired: 1 out]
  n3 = call <vilib>:"OpenHandle.vi"() -> ("client handle out"=w20:T1)  [unwired: 14 in, 1 out]
  n4 = Close Variable Connection(8:w13, 11:w14) -> ()  [unwired: 1 out]
  n5 = control-ref of="Status"() -> (w2:refnum<vi>)
  n6 = call <vilib>:"AddHeader.vi"("client handle"=w20, "header"="Authorization", "value"=w12) -> ("client handle out"=w19:T1, "error out"=w9:errorcluster)  [unwired: 11 in]
  n7 = property on="Property Node" class="Str"(reference=w2, error in=w9, "Value"="Requesting") -> (reference out=w4:refnum<vi>, error out=w6:errorcluster)
  n8 = property on="Property Node" class="Str"(reference=w4, error in=w6, "Blinking"=TRUE ("Value")) -> (error out=w5:errorcluster)  [unwired: 1 out]
  n9 = call <vilib>:"GET.vi"("client handle"=w19, "url"="https://app.asana.com/api/1.0/tasks?workspace=914676468468&assignee=me", "error in (no error)"=w5, "timeout (10000)"=120000) -> ("headers"=→"Headers":string, "body"=→"Body":string, "error out"=w7:errorcluster)  [unwired: 8 in, 1 out]
  n10 = property on="Property Node" class="Str"(reference=w2, error in=w7, "Value"="Idle") -> ()  [unwired: 2 out]
